vi "Get Children Recursively.vi"(8 "error in (no error)":errorcluster, 11 "Data Item in":refnum<class "Data Item.lvclass">) -> (0 "error out":errorcluster, 2 "Children":refnum<class "Data Item.lvclass">[](array[class]), 3 "Data Item out":refnum<class "Data Item.lvclass">)   [LabVIEW 2020, in "VILab.lvlib" / "Data Item.lvclass"]
uses:
  Data Item.lvclass
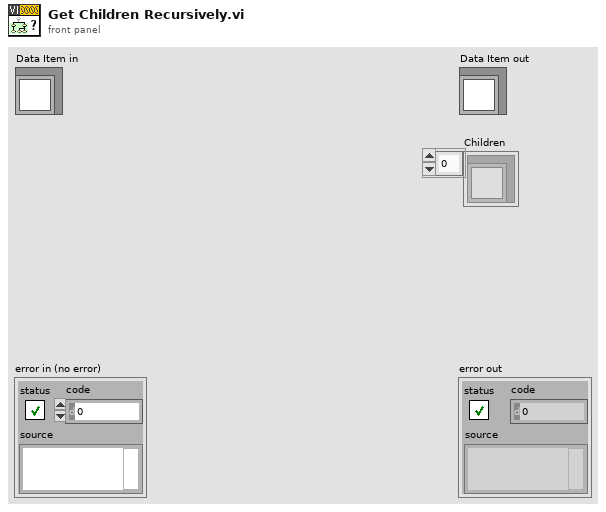
[diagram p1: front panel]
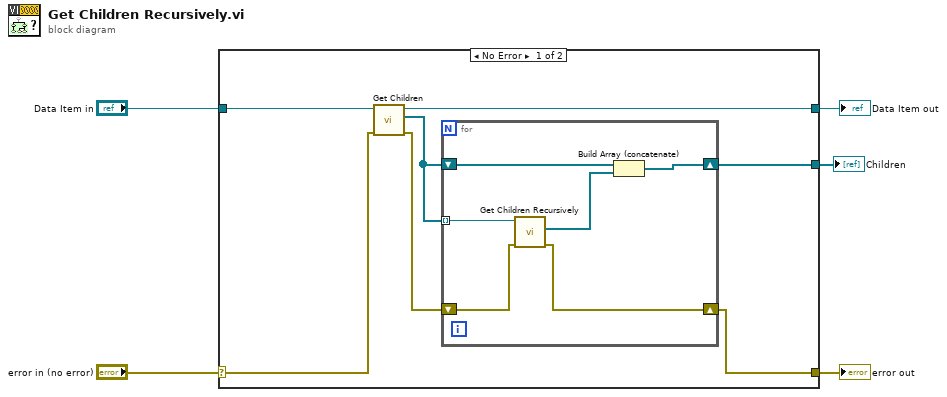
[diagram p0: block diagram]
diagram:
  n1 = case shown="No Error" "error in (no error)" {
    selector: "error in (no error)" -> [w10 w20]
    tunnel: [w6 w20] -> w4
    tunnel: [w11 w19] -> w2
    tunnel: "Data Item in" -> [w12 w19]
    tunnel: [w7 _] -> w1
    frame No Error {
      n2 = call-dynamic "Get Children.vi"("error in (no error)"=w10, "Data Item in"=w12) -> ("error out"=w9:errorcluster, "Children"=w8:refnum<class "Data Item.lvclass">[], "Data Item out"=w11:refnum<class "Data Item.lvclass">)  [unwired: 7 in]
      n3 = for {
        tunnel: w8 -> [w18] mode=indexing
        shift-right: [w16] -> w6
        shift-left: w9 -> [w17]
        shift-right: [w13] -> w7
        shift-left: w8 -> [w15]
        n4 = call "Get Children Recursively.vi"("error in (no error)"=w17, "Data Item in"=w18) -> ("error out"=w16:errorcluster, "Children"=w14:refnum<class "Data Item.lvclass">[])  [unwired: 7 in, 1 out]
        n5 = Build Array (concatenate)(w15, w14) -> (w13:refnum<class "Data Item.lvclass">[])
      }
    }
    frame Error {
    }
  }
  "error out" <- w4
  "Data Item out" <- w2
  "Children" <- w1
